vi "ReadMaxAmp.vi"(8 "error in (no error)":errorcluster, 9 "Channel":dbl, 11 "PXIe 5185 in":refnum<class "PXIe 5185.lvclass">) -> (0 "error out":errorcluster, 1 "Amplitude":dbl, 3 "PXIe 5185 out":refnum<class "PXIe 5185.lvclass">)   [LabVIEW 2015, in "PXIe 5185.lvclass"]
uses:
  PXIe 5185.lvclass
  <userlib>/Common Components/Hardware/Scope/Scope.lvclass
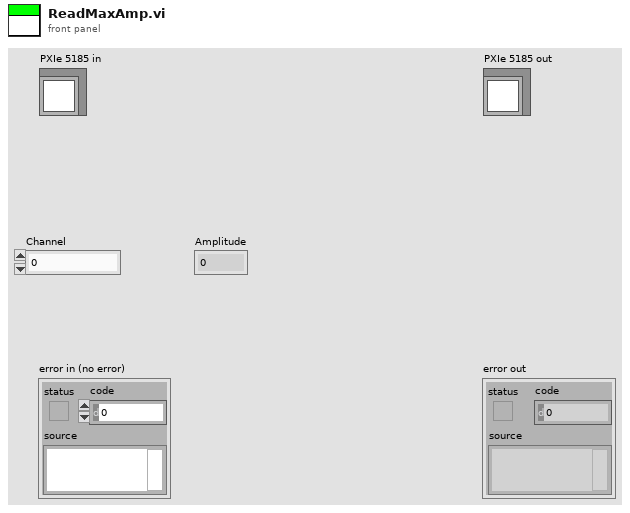
[diagram p1: front panel]
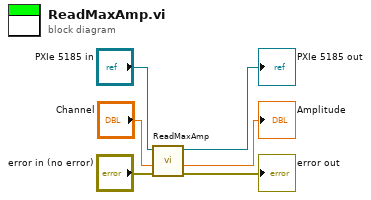
[diagram p0: block diagram]
diagram:
  n1 = call-parent "ReadMaxAmp.vi"("error in (no error)"="error in (no error)", "Channel"="Channel", "Scope in"="PXIe 5185 in") -> ("error out"=→"error out":errorcluster, "Amplitude"=→"Amplitude":dbl, "Scope out"=→"PXIe 5185 out":refnum<class "PXIe 5185.lvclass">)  [unwired: 6 in]
